vi "Readable String.vi"(11 "HighLimit Condition in":refnum<class "HighLimit Condition.lvclass">) -> (2 "String":string)   [LabVIEW 2020, in "VolatusSeq.lvlib" / "HighLimit Condition.lvclass"]
uses:
  HighLimit Condition.lvclass
  HighLimit Condition.lvclass/HighLimit Condition.ctl
  lv-vecto/Vecto/Channel DBL/Channel DBL.lvclass/Channel DBL.ctl
  lv-vecto/Vecto/Group DBL/Group DBL.lvclass
  C:/dev/lv20CE/relink/lv-vecto/Vecto/Group/Group.lvclass
  lv-vecto/Vecto/Group/Channel Info by Index.vi
  Condition Value/Condition Value.lvclass
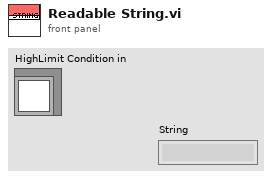
[diagram p1: front panel]
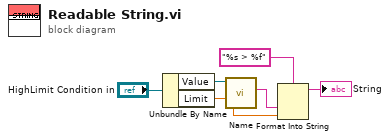
[diagram p0: block diagram]
diagram:
  n1 = Unbundle By Name("HighLimit Condition in") -> ("Value"=w2:refnum<class "Condition Value.lvclass">, "Limit"=w6:dbl)
  n2 = call "Name.vi"("Condition Value in"=w2) -> ("Name"=w1:string)  [unwired: 10 in]
  n3 = Format Into String(format string="%s > %f", w1, w6) -> (resulting string=→"String":string)  [unwired: 2 in, 1 out]
